vi "Teleop.vi"(10 "Match Info":T1={"Autonomous Elapsed Seconds"=0.0, "TeleOp Elapsed Seconds"=0.0, "Disabled Elapsed Seconds"=0.0, "Visited Autonomous"=FALSE, "Visited TeleOp"=FALSE, "Visited Disabled"=FALSE, "Autonomous Settings"={"Autonomous Style"=enum."Independent", "VI Refnum"=refnum}}, 11 "Call Context":T2) -> ()   [LabVIEW 2018]
doc: "This VI is called for each TeleOp packet received from the DS where the robot is not disabled. It is often used to read from the joysticks and update I/O or to update setpoints for timed control loops. It should complete and return within 20 milliseconds or it may miss DS packets."
uses:
  <vilib>/Rock Robotics/WPI/DriverStation/WPI_DriverStationDerivedRobotMode.ctl
  <vilib>/Rock Robotics/WPI/DriverStation/WPI_DriverStationMatch Info.ctl
  <vilib>/Rock Robotics/WPI/Solenoid/WPI_SolenoidValue.ctl
  <vilib>/Rock Robotics/WPI/ThirdParty/Phoenix-LabVIEW/Motor Controller/Controls/CTRE_Phoenix_MotorControl_ControlMode.ctl
  <vilib>/Rock Robotics/WPI/Utilities/WPI_GetSetVariantRefNum.vi
  <vilib>/Rock Robotics/Network Tables/NT Write Boolean Array.vi
  <vilib>/Rock Robotics/Network Tables/NT Write Numeric Array.vi
  <vilib>/Rock Robotics/Network Tables/NT Read Boolean.vi
  <vilib>/Rock Robotics/Network Tables/NT Read Number.vi
  <vilib>/Rock Robotics/WPI/Solenoid/WPI_SolenoidSetEnum.vi
panel:
  out "Enabled":bool
  out "Compressor Running":bool
  out "Sample Slider 0":dbl(slide) scale=0.0..5.0
  out "Sample Boolean 1":bool
  out "Sample Boolean 0":bool
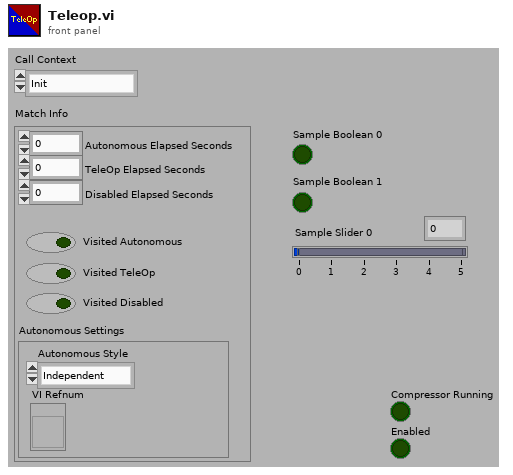
[diagram p1: front panel]
types:
  T1 = typedef "WPI_DriverStationMatch Info.ctl" = cluster{"Autonomous Elapsed Seconds":dbl, "TeleOp Elapsed Seconds":dbl, "Disabled Elapsed Seconds":dbl, "Visited Autonomous":bool, "Visited TeleOp":bool, "Visited Disabled":bool, "Autonomous Settings":cluster{"Autonomous Style":enum16{"Iterative", "Independent"}, "VI Refnum":refnum<vi>}}
  T2 = typedef "WPI_DriverStationDerivedRobotMode.ctl" = enum16{"Init", "Execute", "Stop"}
  T3 = typedef "CTRE_Phoenix_MotorControl_ControlMode.ctl" = u16
  T4 = typedef "WPI_SolenoidValue.ctl" = enum16{"Off", "On", "Forward", "Reverse"}
  T5 = typedef "WPI_JoystickDevRef.ctl" = cluster{"Device":T6}
  T6 = typedef "WPI_JoystickDeviceEnum.ctl" = enum16{"USB 0", "USB 1", "USB 2", "USB 3", "USB 4", "USB 5"}
  T7 = typedef "WPI_CompressorDevRef.ctl" = cluster{"DevStatus":errorcluster, "Pneumatics Control Module":u8}
  T8 = typedef "WPI_MotorControlDeviceRef.ctl" = cluster{"DeviceStatus":errorcluster, "Type":T9, "PWM":cluster{"PWM Channel":T10, "DeadBand":T11}, "CAN":cluster{"Device Number":u8, "SetOutput VI Ref":variant, "GetOutput VI Ref":variant, "Enable VI Ref":variant, "Disable VI Ref":variant, "Data":variant}, "Invert":bool, "DIO PWM":cluster{"PWM \"Enable\" Channel":T10, "DIOChannel":T12, "PWM Rate":dbl}}
  T9 = typedef "WPI_MotorControlType.ctl" = enum16{"PWM", "CAN", "DIO PWM"}
  T10 = typedef "FPGA_DIOPWMChannel.ctl" = enum8{"PWM 0", "PWM 1", "PWM 2", "PWM 3", "PWM 4", "PWM 5", "PWM 6", "PWM 7", "PWM 8", "PWM 9", "PWM MXP 0", "PWM MXP 1", "PWM MXP 2", "PWM MXP 3", "PWM MXP 4", "PWM MXP 5", "PWM MXP 6", "PWM MXP 7", "PWM MXP 8", "PWM MXP 9", "Invalid"}
  T11 = typedef "WPI_PWMDeadband.ctl" = cluster{"Name":string, "maxPositivePwm":i32, "minPositivePwm":i32, "centerPwm":i32, "maxNegativePwm":i32, "minNegativePwm":i32, "angularRange":u16}
  T12 = typedef "FPGA_DIOChannel.ctl" = enum8{"DIO 0", "DIO 1", "DIO 2", "DIO 3", "DIO 4", "DIO 5", "DIO 6", "DIO 7", "DIO 8", "DIO 9", "DIO MXP 0", "DIO MXP 1", "DIO MXP 2", "DIO MXP 3", "DIO MXP 4", "DIO MXP 5", "DIO MXP 6", "DIO MXP 7", "DIO MXP 8", "DIO MXP 9", "DIO MXP 10", "DIO MXP 11", "DIO MXP 12", "DIO MXP 13", "DIO MXP 14", "DIO MXP 15", "SPI Port CS1", "SPI Port CS2", "SPI Port CS3", "SPI Port MISO", "SPI Port MOSI", "Invalid"}
  T13 = typedef "WPI_SolenoidDevRef.ctl" = cluster{"DevStatus":errorcluster, "Pneumatics Control Module":u8, "Forward Solenoid Channel":T14, "Reverse Solenoid Channel":T14}
  T14 = typedef "WPI_SolenoidChannel.ctl" = enum8{"Solenoid 0", "Solenoid 1", "Solenoid 2", "Solenoid 3", "Solenoid 4", "Solenoid 5", "Solenoid 6", "Solenoid 7", "Invalid"}
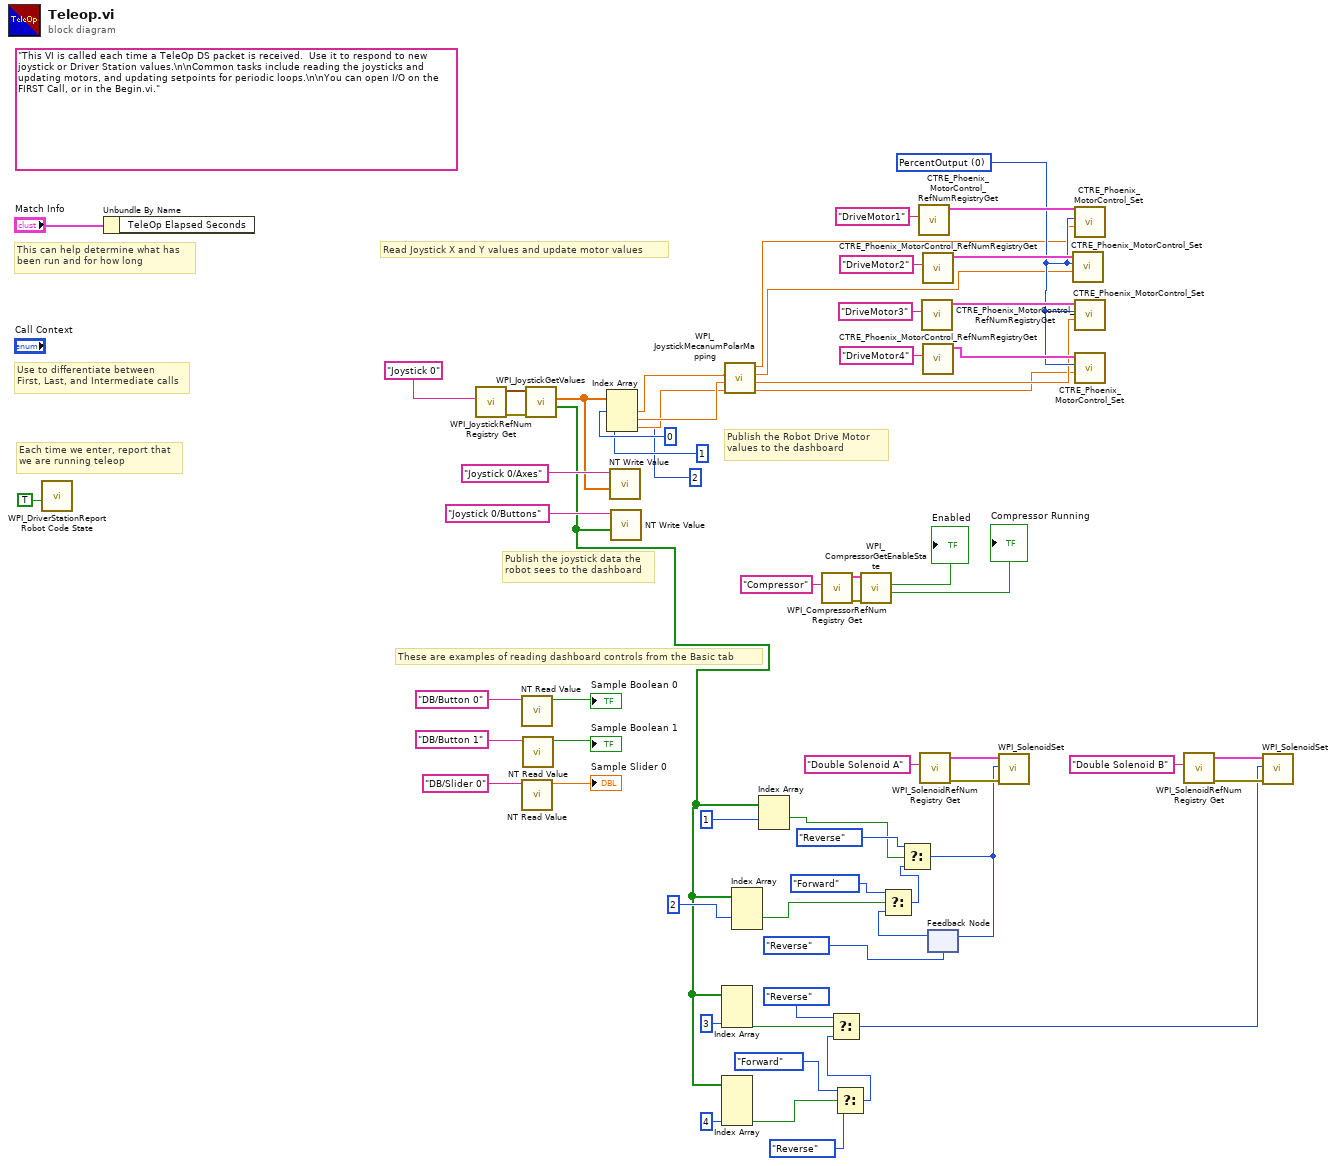
[diagram p0: block diagram]
diagram:
  w10 = T3 0 items=["PercentOutput"=0, "Position"=1, "Velocity"=2, "Current"=3, "Follower"=5, "MotionProfile"=6, "MotionMagic"=7, "MotionProfileArc"=10, "Disabled"=15] ("Control Mode")
  (unwired) "This VI is called each time a TeleOp DS packet is received.  Use it to respond to new joystick or Driver Station values.\n\nCommon tasks include reading the joysticks and updating motors, and updating setpoints for periodic loops.\n\nYou can open I/O on the FIRST Call, or in the Begin.vi."
  # "These are examples of reading dashboard controls from the Basic tab"
  # "Publish the Robot Drive Motor\nvalues to the dashboard"
  # "Publish the joystick data the\nrobot sees to the dashboard"
  # "Each time we enter, report that\nwe are running teleop"
  # "Use to differentiate between\nFirst, Last, and Intermediate calls"
  # "This can help determine what has\nbeen run and for how long"
  # "Read Joystick X and Y values and update motor values"
  n1 = call <vilib>:"WPI_DriverStationReport Robot Code State.vi"("TeleOp"=TRUE ("Autonomous")) -> ()  [unwired: 10 in, 1 out]
  n2 = Unbundle By Name("Match Info") -> ()  [unwired: 1 out]
  n3 = call <vilib>:"WPI_JoystickRefNum Registry Get.vi"("refnum name"="Joystick 0") -> ("error out"=w9:errorcluster, "JoystickDevRef"=w62:T5)  [unwired: 1 in, 8 out]
  n4 = call-poly <vilib>:"NT Read Value.vi"("Name"="DB/Button 0" ("refnum name")) -> ("Boolean"=→"Sample Boolean 0":bool)  [unwired: 9 in, 1 out]
  n5 = call-poly <vilib>:"NT Read Value.vi"("Name"="DB/Slider 0" ("refnum name")) -> ("Numeric"=→"Sample Slider 0":dbl)  [unwired: 9 in, 1 out]
  n6 = call-poly <vilib>:"NT Read Value.vi"("Name"="DB/Button 1" ("refnum name")) -> ("Boolean"=→"Sample Boolean 1":bool)  [unwired: 9 in, 1 out]
  n7 = call <vilib>:"WPI_JoystickGetValues.vi"("error in (no error)"=w9, "JoystickDevRef"=w62) -> ("Buttons"=w19:bool[], "Axes"=w58:dbl[])  [unwired: 5 in, 3 out]
  n8 = Index Array(array=w58, index #1=0 ("index"), index #2=1 ("index"), index #3=2 ("index")) -> (element #1=w8:dbl, element #2=w7:dbl, element #3=w6:dbl)
  n9 = call-poly <vilib>:"NT Write Value.vi"("Numeric Array"=w58, "Name"="Joystick 0/Axes") -> ()  [unwired: 9 in, 1 out]
  n10 = call-poly <vilib>:"NT Write Value.vi"("Boolean Array"=w19, "Name"="Joystick 0/Buttons") -> ()  [unwired: 9 in, 1 out]
  n11 = Index Array(array=w19, index #3=3 ("index")) -> (element #3=w26:bool)  [unwired: 2 in, 2 out]
  n12 = Index Array(array=w19, index #4=4 ("index")) -> (element #4=w21:bool)  [unwired: 3 in, 3 out]
  n13 = call <vilib>:"WPI_JoystickMecanumPolarMapping.vi"("Rotation"=w6, "Direction"=w7, "Magnitude"=w8) -> ("Rear Right"=w1:dbl, "Rear Left"=w3:dbl, "Front Right"=w2:dbl, "Front Left"=w4:dbl)  [unwired: 5 in]
  n14 = Index Array(array=w19, index #2=2 ("index")) -> (element #2=w33:bool)  [unwired: 2 in, 2 out]
  n15 = Index Array(array=w19, index #1=1 ("index")) -> (element #1=w39:bool)  [unwired: 1 in, 1 out]
  n16 = call <vilib>:"WPI_CompressorRefNum Registry Get.vi"("refnum name"="Compressor") -> ("error out"=w49:errorcluster, "CompressorDevRef"=w48:T7)  [unwired: 9 in]
  n17 = Select(t=WPI_SolenoidValue."Forward" ("Value"), s=w21, f=WPI_SolenoidValue."Reverse" ("Value")) -> (s? t:f=w24:T4)
  n18 = Select(t=WPI_SolenoidValue."Reverse" ("Value"), s=w26, f=w24) -> (s? t:f=w22:T4)
  n19 = call <vilib>:"WPI_CompressorGetEnableState.vi"("error in (no error)"=w49, "CompressorDevRef"=w48) -> ("Compressor Running"=→"Compressor Running":bool, "Enabled"=→"Enabled":bool)  [unwired: 6 in, 2 out]
  n20 = call <vilib>:"CTRE_Phoenix_MotorControl_RefNumRegistryGet.vi"("refnum name"="DriveMotor1") -> ("PhoenixMotorControlDevRef"=w14:T8)  [unwired: 9 in, 1 out]
  n21 = call <vilib>:"WPI_SolenoidRefNum Registry Get.vi"("refnum name"="Double Solenoid A") -> ("error out"=w43:errorcluster, "SolenoidDevRef"=w44:T13)  [unwired: 9 in]
  n22 = call <vilib>:"CTRE_Phoenix_MotorControl_RefNumRegistryGet.vi"("refnum name"="DriveMotor3") -> ("PhoenixMotorControlDevRef"=w12:T8)  [unwired: 9 in, 1 out]
  n23 = call <vilib>:"CTRE_Phoenix_MotorControl_RefNumRegistryGet.vi"("refnum name"="DriveMotor2") -> ("PhoenixMotorControlDevRef"=w11:T8)  [unwired: 9 in, 1 out]
  n24 = call <vilib>:"CTRE_Phoenix_MotorControl_RefNumRegistryGet.vi"("refnum name"="DriveMotor4") -> ("PhoenixMotorControlDevRef"=w13:T8)  [unwired: 9 in, 1 out]
  n25 = feedback #1(WPI_SolenoidValue."Reverse" ("Value")) -> (w37:T4)
  n26 = Select(t=WPI_SolenoidValue."Forward" ("Value"), s=w33, f=w37) -> (s? t:f=w36:T4)
  n27 = Select(t=WPI_SolenoidValue."Reverse" ("Value"), s=w39, f=w36) -> (s? t:f=w29:T4)
  n28 = feedback-in #1(w29) -> ()
  n29 = call-poly <vilib>:"WPI_SolenoidSet.vi"("error in (no error)"=w43, "Value"=w29, "SolenoidDevRef"=w44) -> ()  [unwired: 7 in, 2 out]
  n30 = call <vilib>:"CTRE_Phoenix_MotorControl_Set.vi"("Output"=w2, "Control Mode"=w10, "PhoenixMotorControlDevRef"=w11) -> ()  [unwired: 7 in, 2 out]
  n31 = call <vilib>:"CTRE_Phoenix_MotorControl_Set.vi"("Output"=w4, "Control Mode"=w10, "PhoenixMotorControlDevRef"=w14) -> ()  [unwired: 7 in, 2 out]
  n32 = call <vilib>:"CTRE_Phoenix_MotorControl_Set.vi"("Output"=w3, "Control Mode"=w10, "PhoenixMotorControlDevRef"=w12) -> ()  [unwired: 7 in, 2 out]
  n33 = call <vilib>:"CTRE_Phoenix_MotorControl_Set.vi"("Output"=w1, "Control Mode"=w10, "PhoenixMotorControlDevRef"=w13) -> ()  [unwired: 7 in, 2 out]
  n34 = call <vilib>:"WPI_SolenoidRefNum Registry Get.vi"("refnum name"="Double Solenoid B") -> ("error out"=w31:errorcluster, "SolenoidDevRef"=w32:T13)  [unwired: 9 in]
  n35 = call-poly <vilib>:"WPI_SolenoidSet.vi"("error in (no error)"=w31, "Value"=w22, "SolenoidDevRef"=w32) -> ()  [unwired: 7 in, 2 out]
